vi "GetPixyObjectError.vi"(10 "X Value":dbl) -> (2 "Output":dbl, 5 "Object In Parameters":bool)   [LabVIEW 2016]
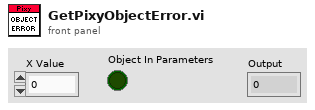
[diagram p1: front panel]
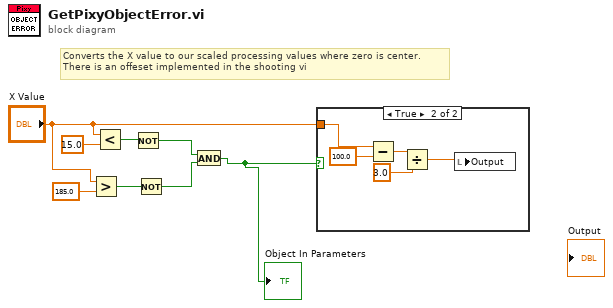
[diagram p0: block diagram]
diagram:
  # "Converts the X value to our scaled processing values where zero is center.\nThere is an offeset implemented in the shooting vi"
  n1 = Greater?(x="X Value", y=185.0) -> (0:w4:bool)
  n2 = Less?(x="X Value", y=15.0) -> (x < y?=w5:bool)
  n3 = Not(x=w5) -> (.not. x?=w3:bool)
  n4 = Not(x=w4) -> (.not. x?=w2:bool)
  n5 = And(x=w3, y=w2) -> (x .and. y?=w1:bool)
  "Object In Parameters" <- w1
  n6 = case shown="True" w1 {
    tunnel: "X Value" -> [_ w13]
    frame False {
    }
    frame True {
      n7 = Subtract(x=w13, y=100.0) -> (x-y=w11:dbl)
      n8 = Divide(x=w11, y=3.0) -> (x/y=w9:dbl)
      n9 = local write "Output"(w9) -> ()
    }
  }
